vi "Configure Banana.vi"(7 "Strategies":T1, 8 "error in":errorcluster, 10 "Peels":refnum<class "BananaPeel.lvclass">[](array[class])) -> (0 "error out":errorcluster, 3 "Variety Configured":string)   [LabVIEW 2021, in "Bananas.lvlib"]
uses:
  Bananas.lvlib
  BananaPeel/BananaPeel.lvclass
  Assertion Strategies -- cluster.ctl
  AssertTrue/AssertTrue.lvclass
  Banana/Banana.lvclass
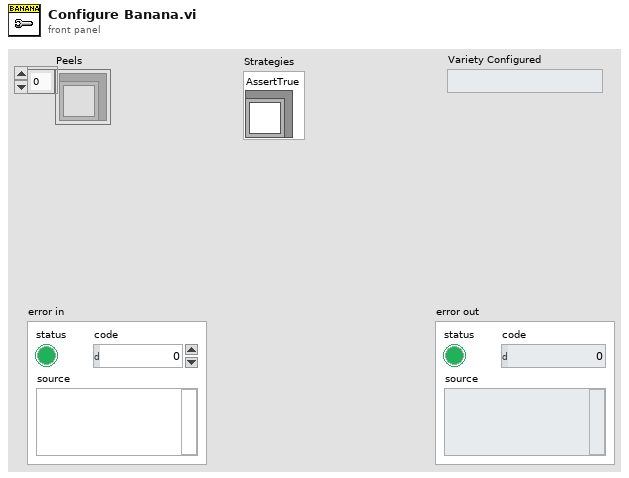
[diagram p1: front panel]
types:
  T1 = typedef "Bananas.lvlib/Assertion Strategies -- cluster.ctl" = cluster{"AssertTrue":refnum<class "AssertTrue.lvclass">}
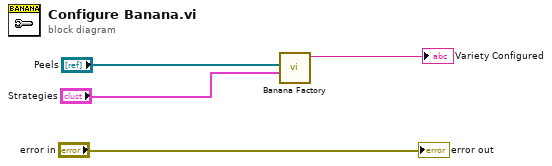
[diagram p0: block diagram]
diagram:
  n1 = call "Banana Factory.vi"("Strategies"="Strategies", "Peels"="Peels") -> ("Variety Configured"=→"Variety Configured":string)  [unwired: 8 in, 1 out]
  "error out" <- "error in"
